vi "createArrayFromComma.vi"(1 "String":string) -> (0 "Array":dbl[](array[numeric]))   [LabVIEW 2015]
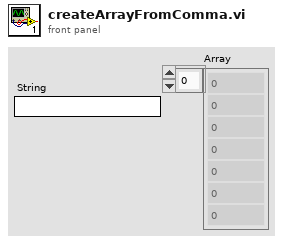
[diagram p1: front panel]
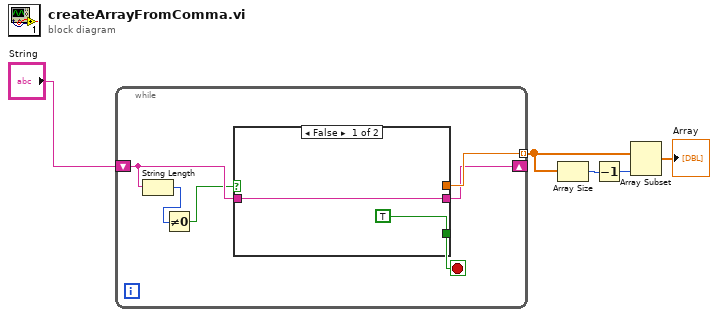
[diagram p0: block diagram]
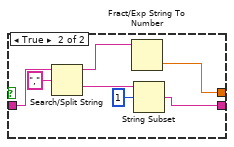
[diagram p2: hidden frame]
diagram:
  n1 = while {
    tunnel: [w11] -> w4 mode=indexing
    shift-right: [w7] -> _
    shift-left: "String" -> [w10]
    stop <- w6 stop-if-true
    n2 = String Length(string=w10) -> (length=w9:i32)
    n3 = Not Equal To 0?(x=w9) -> (x != 0?=w8:bool)
    n4 = case shown="False" w8 {
      tunnel: w10 -> [w13 w20]
      tunnel: [_ w18] -> w11
      tunnel: [w13 w15] -> w7
      tunnel: [TRUE _] -> w6
      frame False {
      }
      frame True {
        n5 = Search/Split String(string=w20, search string/char (-)=",") -> (substring before match=w19:string, match + rest of string=w17:string)  [unwired: 1 in, 1 out]
        n6 = Fract/Exp String To Number(string=w19) -> (number=w18:dbl)  [unwired: 3 in, 1 out]
        n7 = String Subset(string=w17, offset (0)=1) -> (substring=w15:string)  [unwired: 1 in]
      }
    }
  }
  n8 = Array Size(array=w4) -> (size(s)=w3:i32)
  n9 = Decrement(x=w3) -> (x-1=w2:i32)
  n10 = Array Subset(array=w4, length=w2) -> (→"Array":dbl[])  [unwired: 1 in]
